vi "Get Random Background.vi"() -> (3 "Numeric":u16)   [LabVIEW 2021, in "Game.lvclass"]
uses:
  Game.lvclass
  <vilib>/numeric/Random Number (Range) DBL.vi
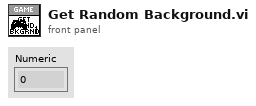
[diagram p1: front panel]
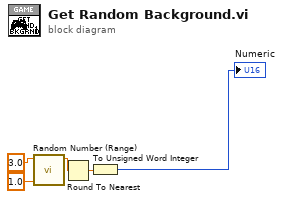
[diagram p0: block diagram]
diagram:
  n1 = call-poly <vilib>:"Random Number (Range).vi"("lower bound (0)"=1.0 ("Low"), "upper bound (100)"=3.0 ("High")) -> ("number"=w3:dbl)  [unwired: 9 in]
  n2 = Round To Nearest(number=w3) -> (nearest integer value=w4:dbl)
  n3 = To Unsigned Word Integer(number=w4) -> (unsigned 16bit integer=→"Numeric":u16)
